vi "Write Customer A's Enqueuer.vi"(8 "error in (no error)":errorcluster, 10 "Customer's A Queue":refnum<class "Message Enqueuer.lvclass">, 11 "ShopAssistant in":refnum<class "ShopAssistant.lvclass">) -> (0 "error out":errorcluster, 3 "ShopAssistant out":refnum<class "ShopAssistant.lvclass">)   [LabVIEW 2020, in "ShopAssistant.lvlib" / "ShopAssistant.lvclass"]
uses:
  ShopAssistant.lvclass
  <vilib>/ActorFramework/Message Enqueuer/Message Enqueuer.lvclass
  ShopAssistant.lvclass/ShopAssistant.ctl
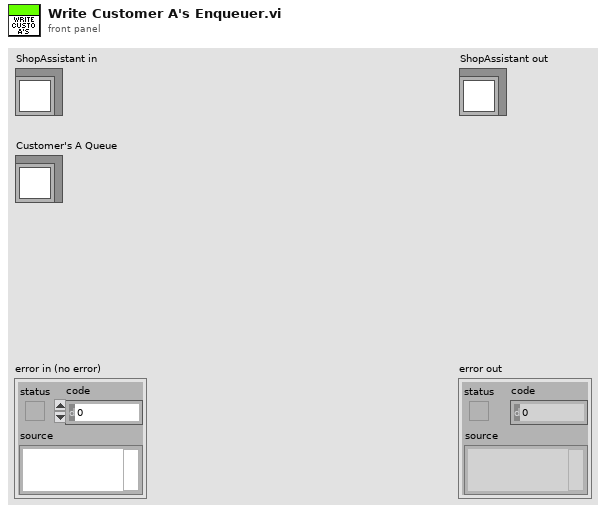
[diagram p1: front panel]
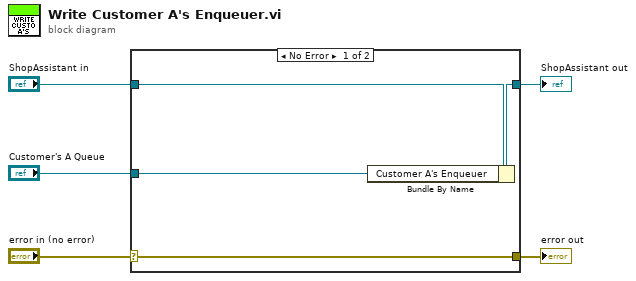
[diagram p0: block diagram]
diagram:
  n1 = case shown="No Error" "error in (no error)" {
    selector: "error in (no error)" -> [w9 w10]
    tunnel: [w9 w10] -> w4
    tunnel: [w7 w11] -> w2
    tunnel: "ShopAssistant in" -> [w8 w11]
    tunnel: "Customer's A Queue" -> [w6 _]
    frame No Error {
      n2 = Bundle By Name(cluster=w8, "Customer A's Enqueuer"=w6) -> (w7:refnum<class "ShopAssistant.lvclass">)
    }
    frame Error {
    }
  }
  "error out" <- w4
  "ShopAssistant out" <- w2
